vi "Read errors mMc.vi"(1 "Port":T1={"P type"=0, "reference"="", " Terminator "="\r\n", "Timeout"=300} {"Timeout" step=10; "P type" items=["none", "RS-232C"]}, 3 "error in (no error)":errorcluster, 5 "Controller #":string) -> (7 "errors":string, 9 "error out":errorcluster)   [LabVIEW 2015]
doc: "ERR 命令：读取并清除错误"
panel:
  # "Read errors"
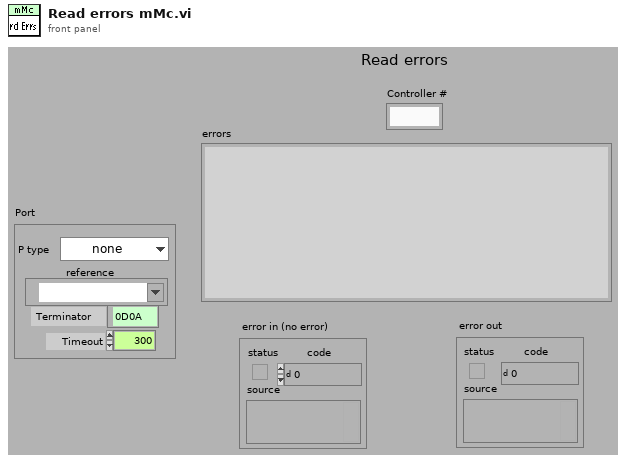
[diagram p1: front panel]
types:
  T1 = cluster{"P type":u16, "reference":refnum<visa-resource-name>, " Terminator ":string, "Timeout":i32}
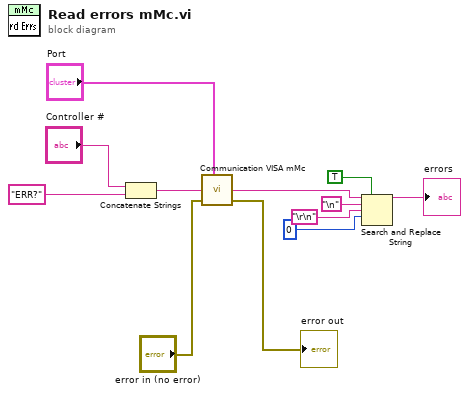
[diagram p0: block diagram]
diagram:
  n1 = Concatenate Strings("Controller #", "ERR?") -> (w8:string)
  n2 = call <instrlib>:"Communication VISA mMc.vi"("Port"="Port", "Command"=w8, "error in (no error)"="error in (no error)") -> ("Return"=w6:string, "error out"=→"error out":errorcluster)  [unwired: 3 in, 2 out]
  n3 = Search and Replace String(replace all?=TRUE ("replace all? (F)"), input string=w6, search string="\n", replace string="\r\n", offset=0 ("offset past replacement")) -> (result string=→"errors":string)  [unwired: 3 in, 3 out]
